vi "Ex4.vi"() -> ()   [LabVIEW 2016]
uses:
  <vilib>/Utility/file.llb/Read Delimited Spreadsheet (DBL).vi
panel:
  out "결과 값":string
  in  "parameter2":dbl
  in  "parameter 1":dbl
  in  "file path (dialog if empty)":path caption="파일 경로(비었을 경우 대화 상자 창)"
  out "all rows":dbl[][](array[numeric]) caption="모든 행"
  in  "format (%.3f)":string="%.3f" caption="포맷(%.3f)"
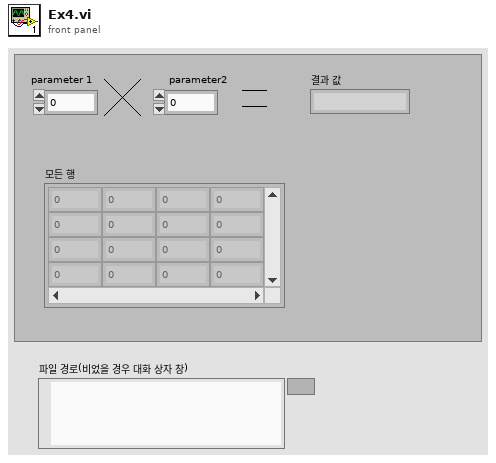
[diagram p1: front panel]
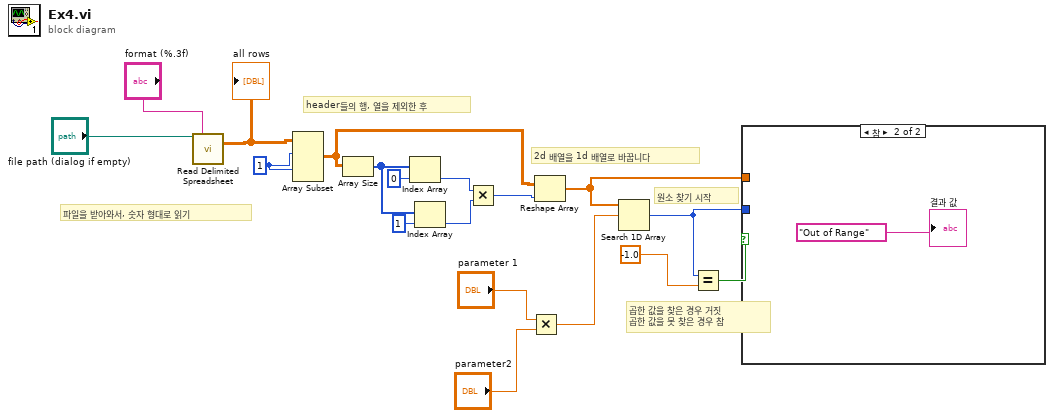
[diagram p0: block diagram]
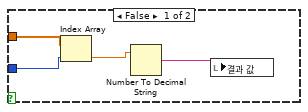
[diagram p2: hidden frame]
diagram:
  w14 = 1
  # "원소 찾기 시작"
  # "2d 배열을 1d 배열로 바꿉니다"
  # "header들의 행, 열을 제외한 후"
  # "곱한 값을 찾은 경우 거짓 \n곱한 값을 못 찾은 경우 참"
  # "파일을 받아와서, 숫자 형대로 읽기"
  n1 = call-poly <vilib>:"Read Delimited Spreadsheet.vi"("file path (dialog if empty)"="file path (dialog if empty)", "format (%.3f)"="format (%.3f)") -> ("all rows"=w7:dbl[][])  [unwired: 8 in, 5 out]
  "all rows" <- w7
  n2 = Array Subset(array=w7, index (row)=w14, index (col)=w14) -> (w6:dbl[][])  [unwired: 2 in]
  n3 = Array Size(array=w6) -> (size(s)=w12:i32[])
  n4 = Index Array(array=w12, index=0 ("인덱스")) -> (element=w10:i32)
  n5 = Index Array(array=w12, index=1 ("인덱스")) -> (element=w9:i32)
  n6 = Multiply(x=w10, y=w9) -> (x*y=w8:i32)
  n7 = Multiply(x="parameter 1", y="parameter2") -> (x*y=w5:dbl)
  n8 = Reshape Array(w6, w8) -> (w2:dbl[])
  n9 = Search 1D Array(1D array=w2, element=w5) -> (index of element=w1:i32)  [unwired: 1 in]
  n10 = Equal?(x=w1, y=-1.0) -> (x = y?=w3:bool)
  n11 = case shown="참" w3 {
    tunnel: w2 -> [w22 _]
    tunnel: w1 -> [w21 _]
    frame False {
      n12 = Index Array(array=w22, index=w21) -> (element=w20:dbl)
      n13 = Number To Decimal String(number=w20) -> (decimal integer string=w19:string)  [unwired: 1 in]
      n14 = local write "결과 값"(w19) -> ()
    }
    frame True {
      "결과 값" <- "Out of Range"
    }
  }
